vi "Multiply Force.vi"(10 "force in":dbl, 11 "Lever in":refnum<class "Lever.lvclass">) -> (2 "force out":dbl)   [LabVIEW 2023, in "Lever.lvclass"]
uses:
  Lever.lvclass
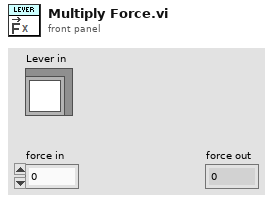
[diagram p1: front panel]
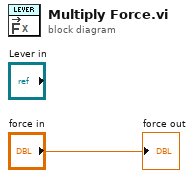
[diagram p0: block diagram]
diagram:
  "force out" <- "force in"
